vi "listen for GFG event - Example.vi"() -> ()   [LabVIEW 2012]
doc: "SciScan 1.2 160622"
panel:
  out "ZOOM":dbl
  out "moveZabs":dbl
  out "moveYabs":dbl
  out "moveXabs":dbl
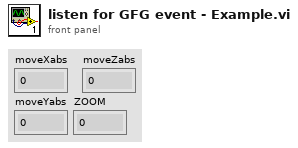
[diagram p1: front panel]
types:
  T1 = cluster{"moveXabs":dbl, "moveYabs":dbl, "moveZabs":dbl}
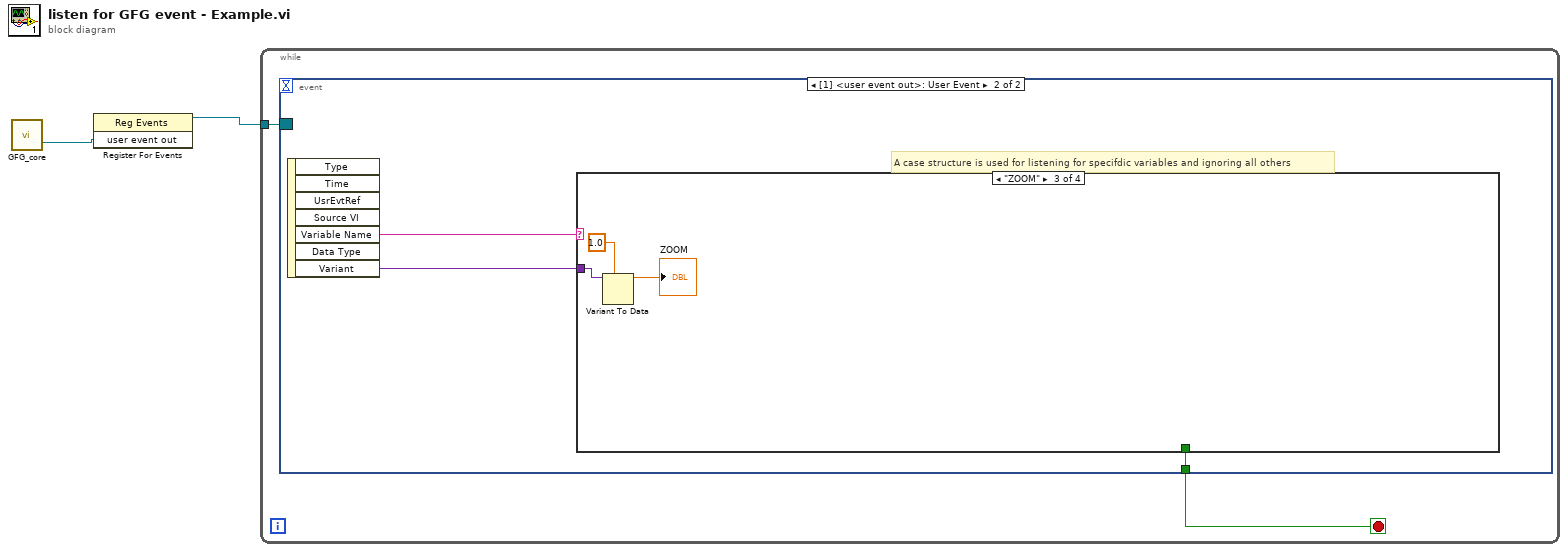
[diagram p0: block diagram]
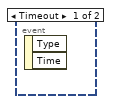
[diagram p2: hidden frame]
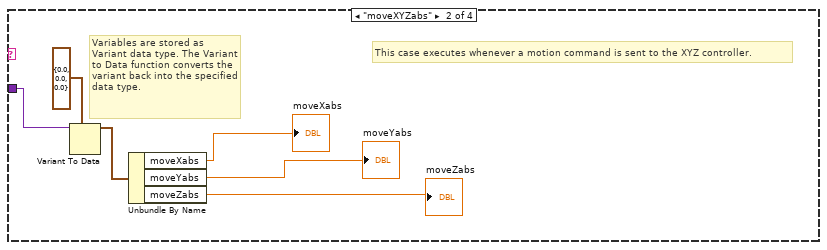
[diagram p4: hidden frame]
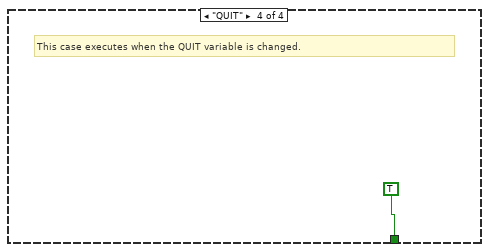
[diagram p5: hidden frame]
diagram:
  n1 = call "GFG_core.vi"() -> ("user event out"=w1:refnum<user-event>)  [unwired: 13 in, 6 out]
  n2 = register-events(w1) -> (reference out=w2:refnum<event-registration>)  [unwired: 2 in, 1 out]
  n3 = while {
    tunnel: w2 -> [w4]
    stop <- w3 stop-if-true
    n4 = event shown="[1] <user event out>: User Event" {
      selector: w4 -> [_ _]
      dyn-events: _ -> [_ _]
      timeout: _ -> [_ _]
      tunnel: [_ w5] -> w3
      event Timeout {
        n5 = event-data() -> ()  [unwired: 1 in, 2 out]
      }
      event User Event {
        # "A case structure is used for listening for specifdic variables and ignoring all others"
        n6 = event-data() -> ("Variable Name"=w7:string, "Variant"=w6:variant)  [unwired: 1 in, 5 out]
        n7 = case shown="\"ZOOM\"" w7 {
          tunnel: w6 -> [_ w13 w16 _]
          tunnel: [_ _ _ TRUE] -> w5
          frame "False", Default {
          }
          frame "moveXYZabs" {
            # "This case executes whenever a motion command is sent to the XYZ controller."
            # "Variables are stored as Variant data type. The Variant to Data function converts the variant back into the specified data type."
            n8 = Variant To Data(type=T1 {"moveXabs"=0.0, "moveYabs"=0.0, "moveZabs"=0.0} ("output cluster"), Variant=w13) -> (data=w11:T1)  [unwired: 1 in, 1 out]
            n9 = Unbundle By Name(w11) -> ("moveXabs"=→"moveXabs":dbl, "moveYabs"=→"moveYabs":dbl, "moveZabs"=→"moveZabs":dbl)
          }
          frame "ZOOM" {
            n10 = Variant To Data(type=1.0 ("ZOOM"), Variant=w16) -> (data=→"ZOOM":dbl)  [unwired: 1 in, 1 out]
          }
          frame "QUIT" {
            # "This case executes when the QUIT variable is changed."
          }
        }
      }
    }
  }
